vi "iBs.vi"(0 "Laser On/Off":bool=TRUE, 1 "VISA resource name":refnum<visa-resource-name>="COM4") -> ()   [LabVIEW 2016]
uses:
  <vilib>/Instr/_visa.llb/VISA Configure Serial Port (Instr).vi
panel:
  in  "Laser On/Off 2":bool=TRUE
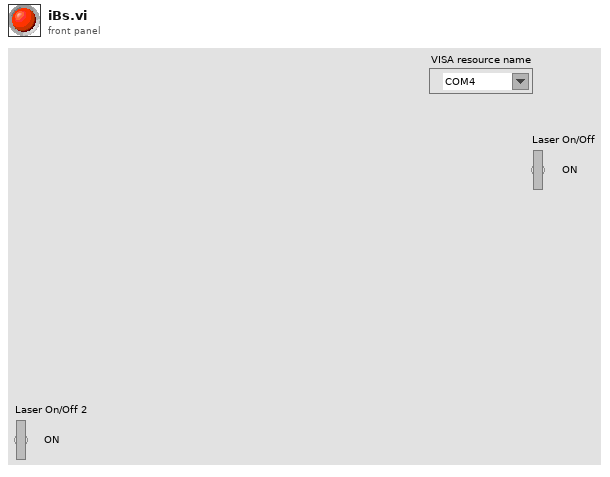
[diagram p1: front panel]
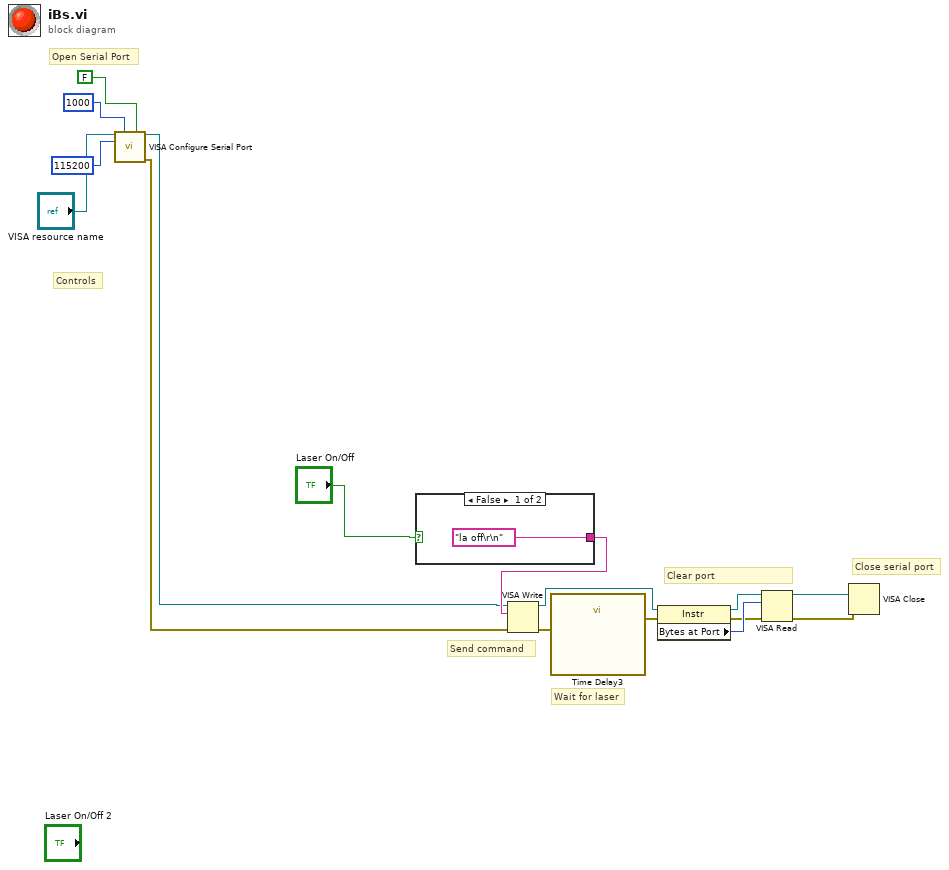
[diagram p0: block diagram]
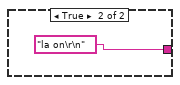
[diagram p2: hidden frame]
diagram:
  # "Close serial port"
  # "Clear port"
  # "Wait for laser"
  # "Send command"
  # "Controls"
  # "Open Serial Port"
  n1 = call-poly "VISA Configure Serial Port"("VISA resource name"="VISA resource name", "timeout (10sec)"=u32 1000, "Enable Termination\nChar (T)"=FALSE ("Enable Termination\nChar (T)"), "baud rate (9600)"=u32 115200) -> ("VISA resource name out"=w5:refnum<visa-resource-name>, "error out"=w4:errorcluster)  [unwired: 10 in]
  n2 = case shown="False" "Laser On/Off" {
    tunnel: ["la off\r\n" "la on\r\n"] -> w6
    frame False {
    }
    frame True {
    }
  }
  n3 = VISA Write(VISA resource name=w5, write buffer=w6, error in (no error)=w4) -> (VISA resource name out=w7:refnum<visa-resource-name>, error out=w9:errorcluster)  [unwired: 1 out]
  n4 = call "Time Delay3"("error in (no error)"=w9) -> ("error out"=w8:errorcluster)  [unwired: 10 in]
  n5 = property class="Instr"(reference=w7, error in=w8) -> (reference out=w12:refnum<visa-resource-name>, error out=w10:errorcluster, "Bytes at Port"=w11:u32)
  n6 = VISA Read(VISA resource name=w12, byte count=w11, error in (no error)=w10) -> (VISA resource name out=w3:refnum<visa-resource-name>, error out=w2:errorcluster)  [unwired: 2 out]
  n7 = VISA Close(VISA resource name=w3, error in (no error)=w2) -> ()  [unwired: 1 out]
